vi "Teleop.vi"(10 "Match Info":T1={"Autonomous Elapsed Seconds"=0.0, "TeleOp Elapsed Seconds"=0.0, "Disabled Elapsed Seconds"=0.0, "Visited Autonomous"=FALSE, "Visited TeleOp"=FALSE, "Visited Disabled"=FALSE, "Autonomous Settings"={"Autonomous Style"=enum."Independent", "VI Refnum"=refnum}}, 11 "Call Context":T2) -> ()   [LabVIEW 2015]
doc: "This VI is called for each TeleOp packet received from the DS where the robot is not disabled. It is often used to read from the joysticks and update I/O or to update setpoints for timed control loops. It should complete and return within 20 milliseconds or it may miss DS packets."
uses:
  <vilib>/Rock Robotics/WPI/DriverStation/WPI_DriverStationDerivedRobotMode.ctl
  <vilib>/Rock Robotics/WPI/DriverStation/WPI_DriverStationMatch Info.ctl
  <vilib>/Rock Robotics/WPI/Utilities/WPI_GetSetVariantRefNum.vi
  <vilib>/Rock Robotics/Network Tables/NT Write Boolean Array.vi
  <vilib>/Rock Robotics/Network Tables/NT Write Numeric Array.vi
  <vilib>/Rock Robotics/Network Tables/NT Read Boolean.vi
  <vilib>/Rock Robotics/Network Tables/NT Read Number.vi
panel:
  out "Sample Slider 0":dbl(slide) scale=0.0..5.0
  out "Sample Boolean 1":bool
  out "Sample Boolean 0":bool
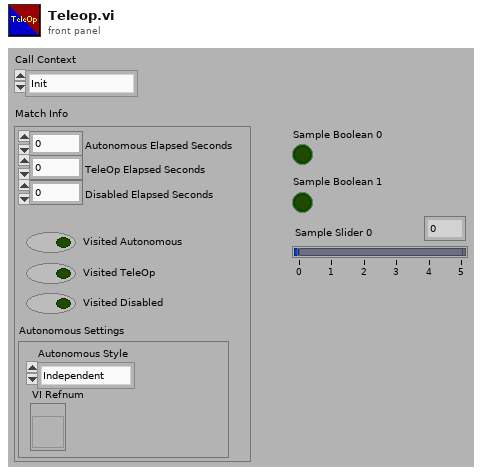
[diagram p1: front panel]
types:
  T1 = typedef "WPI_DriverStationMatch Info.ctl" = cluster{"Autonomous Elapsed Seconds":dbl, "TeleOp Elapsed Seconds":dbl, "Disabled Elapsed Seconds":dbl, "Visited Autonomous":bool, "Visited TeleOp":bool, "Visited Disabled":bool, "Autonomous Settings":cluster{"Autonomous Style":enum16{"Iterative", "Independent"}, "VI Refnum":refnum<vi>}}
  T2 = typedef "WPI_DriverStationDerivedRobotMode.ctl" = enum16{"Init", "Execute", "Stop"}
  T3 = typedef "WPI_JoystickDevRef.ctl" = cluster{"Device":T4}
  T4 = typedef "WPI_JoystickDeviceEnum.ctl" = enum16{"USB 0", "USB 1", "USB 2", "USB 3", "USB 4", "USB 5"}
  T5 = typedef "WPI_RobotDriveDevRef.ctl" = cluster{"DevStatus":errorcluster, "Motors[]":T6[], "Square Inputs":bool, "Max Output":dbl}
  T6 = typedef "WPI_MotorControlDeviceRef.ctl" = cluster{"DeviceStatus":errorcluster, "Type":T7, "PWM":cluster{"PWM Channel":T8, "DeadBand":T9}, "CAN":cluster{"Device Number":u8, "Control Mode":T10, "Semaphore":T11, "Max Vout":dbl, "TalonSRX Control Mode":T12}, "Invert":bool}
  T7 = typedef "WPI_MotorControlType.ctl" = enum16{"PWM", "CAN", "CANTalonSRX"}
  T8 = typedef "FPGA_DIOPWMChannel.ctl" = enum8{"PWM 0", "PWM 1", "PWM 2", "PWM 3", "PWM 4", "PWM 5", "PWM 6", "PWM 7", "PWM 8", "PWM 9", "PWM MXP 0", "PWM MXP 1", "PWM MXP 2", "PWM MXP 3", "PWM MXP 4", "PWM MXP 5", "PWM MXP 6", "PWM MXP 7", "PWM MXP 8", "PWM MXP 9", "Invalid"}
  T9 = typedef "WPI_PWMDeadband.ctl" = cluster{"Name":string, "maxPositivePwm":i32, "minPositivePwm":i32, "centerPwm":i32, "maxNegativePwm":i32, "minNegativePwm":i32, "angularRange":u16}
  T10 = typedef "WPI_CANJaguar_ControlMode.ctl" = enum8{"Percent VBus", "Current", "Speed", "Position", "Voltage"}
  T11 = typedef "Semaphore RefNum" = refnum<k1>
  T12 = typedef "WPI_CANTalonSRX_APIControlMode.ctl" = enum8{"Percent VBus", "Speed", "Position", "Slave", "Unchanged / Invalid", "Voltage Compensation", "Current", "Motion Profile"}
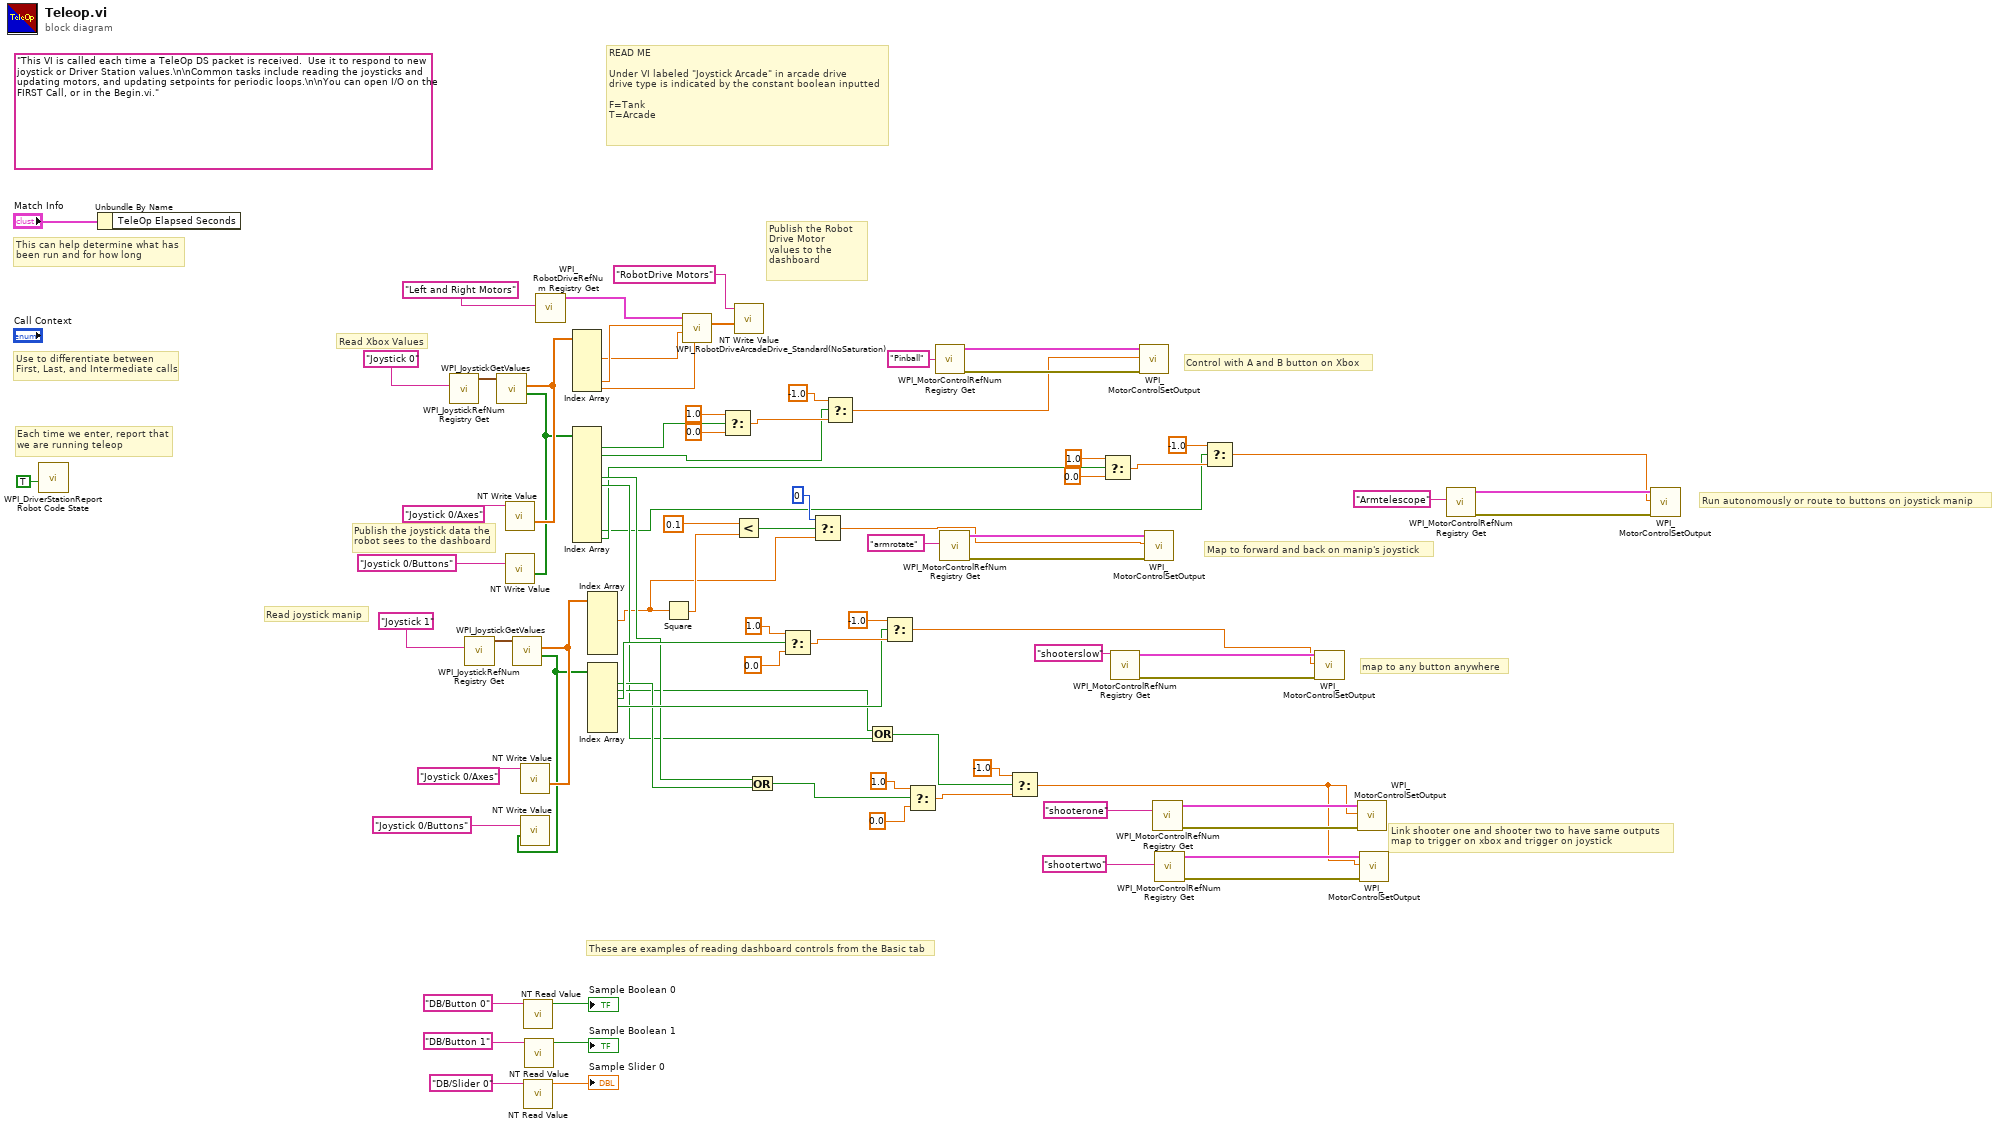
[diagram p0: block diagram]
diagram:
  (unwired) "This VI is called each time a TeleOp DS packet is received.  Use it to respond to new joystick or Driver Station values.\n\nCommon tasks include reading the joysticks and updating motors, and updating setpoints for periodic loops.\n\nYou can open I/O on the FIRST Call, or in the Begin.vi."
  # "map to any button anywhere"
  # "Read joystick manip"
  # "Map to forward and back on manip's joystick"
  # "Run autonomously or route to buttons on joystick manip"
  # "Control with A and B button on Xbox"
  # "Link shooter one and shooter two to have same outputs \nmap to trigger on xbox and trigger on joystick"
  # "READ ME\n\nUnder VI labeled \"Joystick Arcade\" in arcade drive\ndrive type is indicated by the constant boolean inputted\n\nF=Tank\nT=Arcade"
  # "These are examples of reading dashboard controls from the Basic tab"
  # "Publish the Robot Drive Motor\nvalues to the dashboard"
  # "Publish the joystick data the\nrobot sees to the dashboard"
  # "Each time we enter, report that\nwe are running teleop"
  # "Use to differentiate between\nFirst, Last, and Intermediate calls"
  # "This can help determine what has\nbeen run and for how long"
  # "Read Xbox Values"
  n1 = call <vilib>:"WPI_DriverStationReport Robot Code State.vi"("TeleOp"=TRUE ("Autonomous")) -> ()  [unwired: 10 in, 1 out]
  n2 = Unbundle By Name("Match Info") -> ()  [unwired: 1 out]
  n3 = call <vilib>:"WPI_JoystickRefNum Registry Get.vi"("refnum name"="Joystick 0") -> ("JoystickDevRef"=w79:T3)  [unwired: 1 in, 9 out]
  n4 = call <vilib>:"WPI_JoystickRefNum Registry Get.vi"("refnum name"="Joystick 1") -> ("JoystickDevRef"=w61:T3)  [unwired: 1 in, 9 out]
  n5 = call <vilib>:"WPI_JoystickGetValues.vi"("JoystickDevRef"=w79) -> ("Buttons"=w63:bool[], "Axes"=w75:dbl[])  [unwired: 6 in, 3 out]
  n6 = call-poly <vilib>:"NT Write Value.vi"("Numeric Array"=w75, "Name"="Joystick 0/Axes") -> ()  [unwired: 9 in, 1 out]
  n7 = call-poly <vilib>:"NT Write Value.vi"("Boolean Array"=w63, "Name"="Joystick 0/Buttons") -> ()  [unwired: 9 in, 1 out]
  n8 = call <vilib>:"WPI_JoystickGetValues.vi"("JoystickDevRef"=w61) -> ("Buttons"=w27:bool[], "Axes"=w58:dbl[])  [unwired: 6 in, 3 out]
  n9 = call-poly <vilib>:"NT Write Value.vi"("Numeric Array"=w58, "Name"="Joystick 0/Axes") -> ()  [unwired: 9 in, 1 out]
  n10 = call-poly <vilib>:"NT Write Value.vi"("Boolean Array"=w27, "Name"="Joystick 0/Buttons") -> ()  [unwired: 9 in, 1 out]
  n11 = call-poly <vilib>:"NT Read Value.vi"("Name"="DB/Button 0" ("refnum name")) -> ("Boolean"=→"Sample Boolean 0":bool)  [unwired: 9 in, 1 out]
  n12 = call-poly <vilib>:"NT Read Value.vi"("Name"="DB/Slider 0" ("refnum name")) -> ("Numeric"=→"Sample Slider 0":dbl)  [unwired: 9 in, 1 out]
  n13 = call-poly <vilib>:"NT Read Value.vi"("Name"="DB/Button 1" ("refnum name")) -> ("Boolean"=→"Sample Boolean 1":bool)  [unwired: 9 in, 1 out]
  n14 = call <vilib>:"WPI_RobotDriveRefNum Registry Get.vi"("refnum name"="Left and Right Motors") -> ("RobotDriveDevRef"=w81:T5)  [unwired: 1 in, 9 out]
  n15 = Index Array(array=w75) -> (element #2=w64:dbl, element #5=w65:dbl, element #6=w66:dbl)  [unwired: 6 in, 3 out]
  n16 = Index Array(array=w63) -> (element #1=w39:bool, element #2=w35:bool, element #5=w19:bool, element #6=w16:bool, element #12=w1:bool, element #13=w2:bool)  [unwired: 13 in, 7 out]
  n17 = Index Array(array=w58) -> (element #2=w10:dbl)  [unwired: 6 in, 5 out]
  n18 = Index Array(array=w27) -> (element #1=w20:bool, element #2=w17:bool, element #3=w28:bool, element #4=w29:bool)  [unwired: 7 in, 3 out]
  n19 = Square(x=w10) -> (x^2=w12:dbl)
  n20 = call <vilib>:"WPI_RobotDriveArcadeDrive_Standard(NoSaturation).vi"("Numeric"=w66, "Y axis value"=w64, "X axis value"=w65, "RobotDriveDevRef"=w81) -> ("Motor Values"=w68:dbl[])  [unwired: 1 in, 6 out]
  n21 = Select(t=1.0, s=w39, f=0.0) -> (s? t:f=w36:dbl)
  n22 = Less?(x=0.1, y=w12) -> (x < y?=w13:bool)
  n23 = call-poly <vilib>:"NT Write Value.vi"("Numeric Array"=w68, "Name"="RobotDrive Motors") -> ()  [unwired: 9 in, 1 out]
  n24 = Or(x=w19, y=w20) -> (x .or. y?=w18:bool)
  n25 = Select(t=1.0, s=w28, f=0.0) -> (s? t:f=w31:dbl)
  n26 = Select(t=0, s=w13, f=w10) -> (s? t:f=w9:dbl)
  n27 = Select(t=-1.0, s=w35, f=w36) -> (s? t:f=w8:dbl)
  n28 = Or(x=w17, y=w16) -> (x .or. y?=w15:bool)
  n29 = Select(t=-1.0, s=w29, f=w31) -> (s? t:f=w26:dbl)
  n30 = Select(t=1.0, s=w18, f=0.0) -> (s? t:f=w23:dbl)
  n31 = call <vilib>:"WPI_MotorControlRefNum Registry Get.vi"("refnum name"="Pinball") -> ("error out"=w45:errorcluster, "MotorControlDevRef"=w43:T6)  [unwired: 9 in]
  n32 = call <vilib>:"WPI_MotorControlRefNum Registry Get.vi"("refnum name"="armrotate") -> ("error out"=w48:errorcluster, "MotorControlDevRef"=w46:T6)  [unwired: 9 in]
  n33 = Select(t=-1.0, s=w15, f=w23) -> (s? t:f=w21:dbl)
  n34 = Select(t=1.0, s=w2, f=0.0) -> (s? t:f=w5:dbl)
  n35 = call <vilib>:"WPI_MotorControlRefNum Registry Get.vi"("refnum name"="shooterslow") -> ("error out"=w42:errorcluster, "MotorControlDevRef"=w40:T6)  [unwired: 9 in]
  n36 = call <vilib>:"WPI_MotorControlSetOutput.vi"("error in (no error)"=w45, "Output"=w8, "MotorControlDevRef"=w43) -> ()  [unwired: 6 in, 3 out]
  n37 = call <vilib>:"WPI_MotorControlSetOutput.vi"("error in (no error)"=w48, "Output"=w9, "MotorControlDevRef"=w46) -> ()  [unwired: 6 in, 3 out]
  n38 = call <vilib>:"WPI_MotorControlRefNum Registry Get.vi"("refnum name"="shooterone") -> ("error out"=w51:errorcluster, "MotorControlDevRef"=w49:T6)  [unwired: 9 in]
  n39 = call <vilib>:"WPI_MotorControlRefNum Registry Get.vi"("refnum name"="shootertwo") -> ("error out"=w54:errorcluster, "MotorControlDevRef"=w52:T6)  [unwired: 9 in]
  n40 = Select(t=-1.0, s=w1, f=w5) -> (s? t:f=w3:dbl)
  n41 = call <vilib>:"WPI_MotorControlSetOutput.vi"("error in (no error)"=w42, "Output"=w26, "MotorControlDevRef"=w40) -> ()  [unwired: 6 in, 3 out]
  n42 = call <vilib>:"WPI_MotorControlSetOutput.vi"("error in (no error)"=w51, "Output"=w21, "MotorControlDevRef"=w49) -> ()  [unwired: 6 in, 3 out]
  n43 = call <vilib>:"WPI_MotorControlSetOutput.vi"("error in (no error)"=w54, "Output"=w21, "MotorControlDevRef"=w52) -> ()  [unwired: 6 in, 3 out]
  n44 = call <vilib>:"WPI_MotorControlRefNum Registry Get.vi"("refnum name"="Armtelescope") -> ("error out"=w57:errorcluster, "MotorControlDevRef"=w55:T6)  [unwired: 9 in]
  n45 = call <vilib>:"WPI_MotorControlSetOutput.vi"("error in (no error)"=w57, "Output"=w3, "MotorControlDevRef"=w55) -> ()  [unwired: 6 in, 3 out]
